vi "Hands Controller.vi"(8 "error in":errorcluster) -> ()   [LabVIEW 2017]
doc: "This VI executes continuously carrying out the current operation and responding to updates or new operations. It will often contain the timing or control code that is difficult to place directly in TeleOp. This VI generally opens all sensors and motors and isolates the rest of the robot code from knowing how the operations are carried out."
uses:
  <vilib>/Rock Robotics/WPI/Framework/Completion Status.ctl
  Hands Setpoints.ctl
  Hands Operations.ctl
  <vilib>/Rock Robotics/WPI/SafetyOutput/WPI_SafetyOutputConfigMenu.ctl
  <vilib>/Rock Robotics/SystemInterfaces/DIO/FPGA_DIOPWMChannel.ctl
  <vilib>/Rock Robotics/WPI/MotorControl/WPI_MotorControlOpen VictorSP.vi
  <vilib>/Rock Robotics/Network Tables/NT Write Boolean.vi
panel:
  in  "Slide 2":dbl(slide) scale=-0.8..0.8
  in  "Slide":dbl(slide) scale=-0.8..0.8
  out "Waveform Chart":dbl(graph)
  in  "Interactive Values":T1
  out "Current\nCmd":string
  in  "Buttons":cluster{"Execute Cmd":bool, "Abort Cmd":bool}
  out "Command Timing":cluster{"Start Time (ms)":u32, "Iterations":i32}
  out "Status":T3
  # "Tip: It may be helpful to observe inputs and sensor values.\nYou may also want to display tuning or debugging controls."
  # "Interactive Command: You may fill in the settings for a command\nand schedule it with the Execute button. You can observe and abort\nany command while fine tuning the code for the controller."
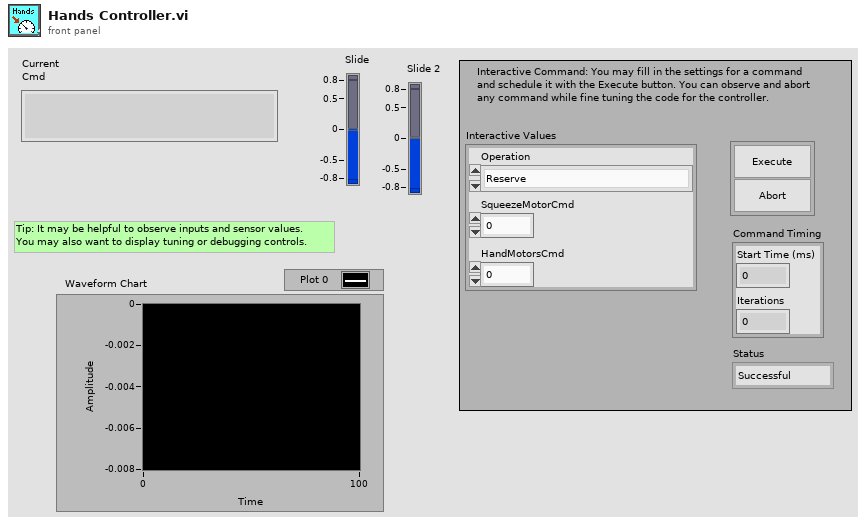
[diagram p1: front panel]
types:
  T1 = typedef "Hands Setpoints.ctl" = cluster{"Operation":T2, "SqueezeMotorCmd":dbl, "HandMotorsCmd":dbl}
  T2 = typedef "Hands Operations.ctl" = enum16{"Reserve", "Read Current", "Immediate"}
  T3 = typedef "Completion Status.ctl" = enum16{"Successful", "Aborted", "Incomplete"}
  T4 = typedef "FPGA_DIOPWMChannel.ctl" = enum8{"PWM 0", "PWM 1", "PWM 2", "PWM 3", "PWM 4", "PWM 5", "PWM 6", "PWM 7", "PWM 8", "PWM 9", "PWM MXP 0", "PWM MXP 1", "PWM MXP 2", "PWM MXP 3", "PWM MXP 4", "PWM MXP 5", "PWM MXP 6", "PWM MXP 7", "PWM MXP 8", "PWM MXP 9", "Invalid"}
  T5 = typedef "WPI_SafetyOutputConfigMenu.ctl" = enum16{"Enable", "Disable"}
  T6 = typedef "WPI_MotorControlDeviceRef.ctl" = cluster{"DeviceStatus":errorcluster, "Type":T7, "PWM":cluster{"PWM Channel":T4, "DeadBand":T8}, "CAN":cluster{"Device Number":u8, "SetOutput VI Ref":variant, "GetOutput VI Ref":variant, "Enable VI Ref":variant, "Disable VI Ref":variant, "Data":variant}, "Invert":bool, "DIO PWM":cluster{"PWM \"Enable\" Channel":T4, "DIOChannel":T9, "PWM Rate":dbl}}
  T7 = typedef "WPI_MotorControlType.ctl" = enum16{"PWM", "CAN", "DIO PWM"}
  T8 = typedef "WPI_PWMDeadband.ctl" = cluster{"Name":string, "maxPositivePwm":i32, "minPositivePwm":i32, "centerPwm":i32, "maxNegativePwm":i32, "minNegativePwm":i32, "angularRange":u16}
  T9 = typedef "FPGA_DIOChannel.ctl" = enum8{"DIO 0", "DIO 1", "DIO 2", "DIO 3", "DIO 4", "DIO 5", "DIO 6", "DIO 7", "DIO 8", "DIO 9", "DIO MXP 0", "DIO MXP 1", "DIO MXP 2", "DIO MXP 3", "DIO MXP 4", "DIO MXP 5", "DIO MXP 6", "DIO MXP 7", "DIO MXP 8", "DIO MXP 9", "DIO MXP 10", "DIO MXP 11", "DIO MXP 12", "DIO MXP 13", "DIO MXP 14", "DIO MXP 15", "SPI Port CS1", "SPI Port CS2", "SPI Port CS3", "SPI Port MISO", "SPI Port MOSI", "Invalid"}
  T10 = typedef "Command Status Info.ctl" = cluster{"Name":string, "Status":T3, "notifier out":T11}
  T11 = typedef "Completion Notifier.ctl" = refnum<notifier>
  T12 = cluster{"Current Command":T1, "Command Timing":cluster{"Start Time (ms)":u32, "Iterations":i32}, "Command Arguments":cluster{"Command Info":T10, "Description":string, "Default Command":T1, "queue out":refnum<queue>, "Subsystem Name":string}}
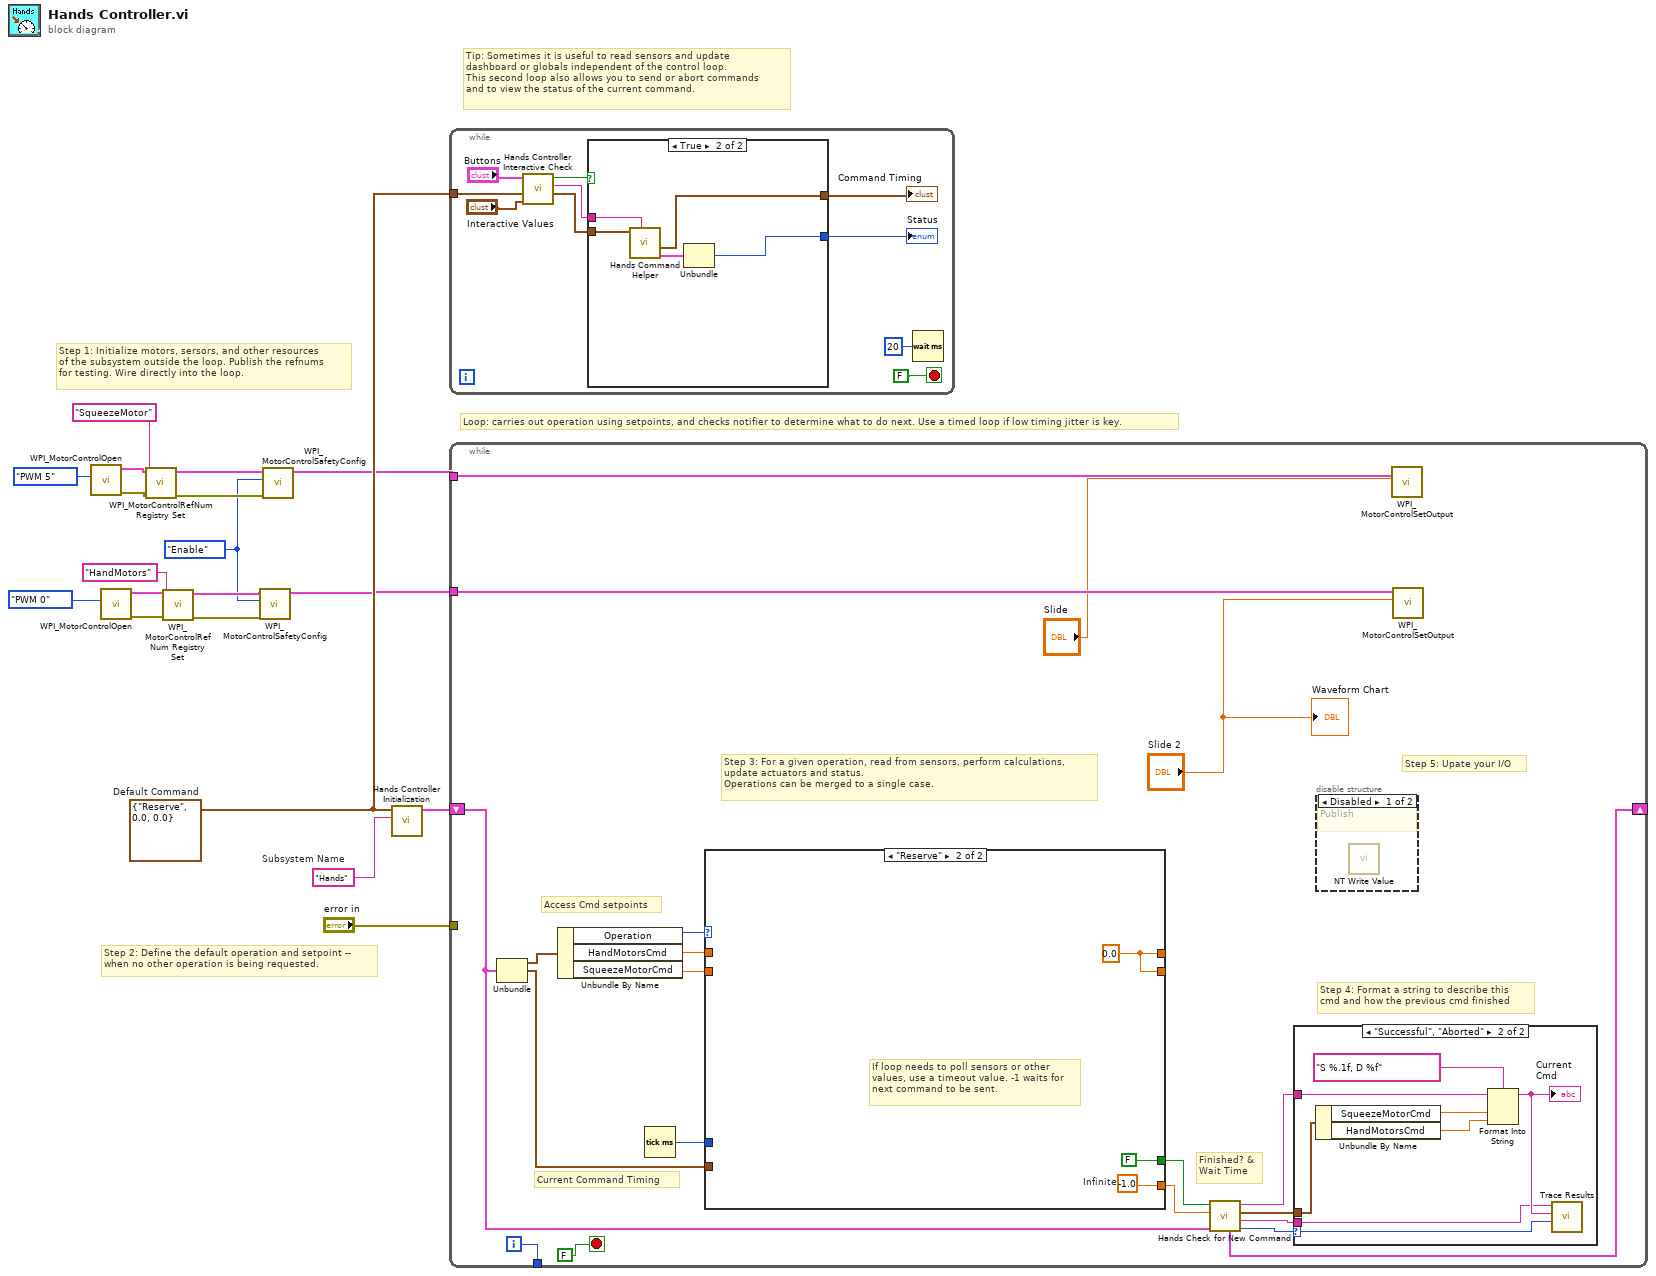
[diagram p0: block diagram]
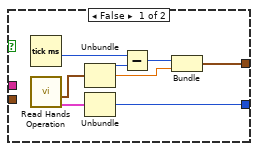
[diagram p2: hidden frame]
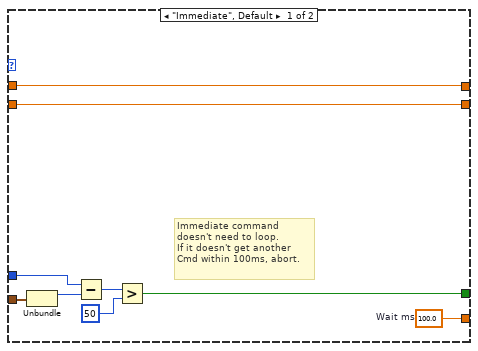
[diagram p5: hidden frame]
diagram:
  w1 = WPI_SafetyOutputConfigMenu."Enable" ("mode")
  w16 = T1 {"Operation"=enum."Reserve", "SqueezeMotorCmd"=0.0, "HandMotorsCmd"=0.0}  # Default Command
  w17 = "Hands"  # Subsystem Name
  # "Tip: Sometimes it is useful to read sensors and update\ndashboard or globals independent of the control loop.\nThis second loop also allows you to send or abort commands\nand to view the status of the current command."
  # "Step 2: Define the default operation and setpoint --\nwhen no other operation is being requested."
  # "Step 1: Initialize motors, sersors, and other resources\nof the subsystem outside the loop. Publish the refnums\nfor testing. Wire directly into the loop."
  # "Loop: carries out operation using setpoints, and checks notifier to determine what to do next. Use a timed loop if low timing jitter is key."
  n1 = call-poly <vilib>:"WPI_MotorControlOpen.vi"("PWM Channel"=FPGA_DIOPWMChannel."PWM 5") -> ("error out"=w7:errorcluster, "MotorControlDeviceRef"=w8:T6)  [unwired: 9 in]
  n2 = call-poly <vilib>:"WPI_MotorControlOpen.vi"("PWM Channel"=FPGA_DIOPWMChannel."PWM 0") -> ("error out"=w12:errorcluster, "MotorControlDeviceRef"=w10:T6)  [unwired: 9 in]
  n3 = call <vilib>:"WPI_MotorControlRefNum Registry Set.vi"("error in (no error)"=w7, "refnum name"="SqueezeMotor", "MotorControlDevRef"=w8) -> ("error out"=w4:errorcluster, "MotorControlDevRef"=w5:T6)  [unwired: 7 in]
  n4 = call <vilib>:"WPI_MotorControlRefNum Registry Set.vi"("error in (no error)"=w12, "refnum name"="HandMotors", "MotorControlDevRef"=w10) -> ("error out"=w13:errorcluster, "MotorControlDevRef"=w14:T6)  [unwired: 7 in]
  n5 = call <vilib>:"WPI_MotorControlSafetyConfig.vi"("error in (no error)"=w13, "mode"=w1, "MotorControlDevRef"=w14) -> ("MotorControlDevRef"=w15:T6)  [unwired: 7 in, 1 out]
  n6 = call <vilib>:"WPI_MotorControlSafetyConfig.vi"("error in (no error)"=w4, "mode"=w1, "MotorControlDevRef"=w5) -> ("MotorControlDevRef"=w3:T6)  [unwired: 7 in, 1 out]
  n7 = call "Hands Controller Initialization.vi"("Subsystem Name"=w17, "Default Command"=w16) -> ("Current Command"=w18:T12)  [unwired: 9 in]
  n8 = while {
    tunnel: w16 -> [w26]
    stop <- FALSE stop-if-true
    n9 = call "Hands Controller Interactive Check.vi"("Interactive Command in"="Interactive Values", "Default Command"=w26, "Buttons"="Buttons") -> ("Interactive Command out"=w23:T1, "Trace String"=w24:string, "Schedule"=w25:bool)  [unwired: 6 in]
    n10 = case shown="True" w25 {
      tunnel: [w37 w42] -> w22
      tunnel: w23 -> [_ w40]
      tunnel: [w33 w38] -> w21
      tunnel: w24 -> [_ w41]
      frame False {
        n11 = Tick Count (ms)() -> (millisecond timer value=w32:u32)
        n12 = call "Read Hands Operation.vi"() -> ("Command Info"=w30:T10, "SubSystem Data"=w31:T1)  [unwired: 9 in, 1 out]
        n13 = Unbundle(w31) -> ("Operation"=w36:T2, "SqueezeMotorCmd"=w34:dbl)  [unwired: 1 out]
        n14 = Unbundle(w30) -> ("Status"=w37:T3)  [unwired: 2 out]
        n15 = Subtract(x=w32, y=w36) -> (x-y=w35:u32)
        n16 = Bundle(w35, "SqueezeMotorCmd"=w34) -> (w33:cluster{u32, "SqueezeMotorCmd":dbl})  [unwired: 1 in]
      }
      frame True {
        n17 = call "Hands Command Helper.vi"("Description"=w41, "SubSystem Data"=w40) -> ("Command Info Out"=w39:T10, "Command Timing"=w38:cluster{"Start Time (ms)":u32, "Iterations":i32})  [unwired: 7 in, 1 out]
        n18 = Unbundle(w39) -> ("Status"=w42:T3)  [unwired: 2 out]
      }
    }
    "Status" <- w22
    "Command Timing" <- w21
    n19 = Wait (ms)(milliseconds to wait=u32 20) -> ()  [unwired: 1 out]
  }
  n20 = while {
    shift-right: [w54] -> _
    shift-left: w18 -> [w47]
    tunnel: [w61] -> _
    tunnel: "error in" -> [_]
    tunnel: w15 -> [w45]
    tunnel: w3 -> [w46]
    i -> [w61]
    stop <- FALSE stop-if-true
    # "Step 5: Upate your I/O"
    # "Step 4: Format a string to describe this\ncmd and how the previous cmd finished"
    # "Current Command Timing"
    # "Access Cmd setpoints"
    # "Finished? &\nWait Time"
    # "Step 3: For a given operation, read from sensors, perform calculations,\nupdate actuators and status.\nOperations can be merged to a single case."
    n21 = Unbundle(w47) -> ("Current Command"=w60:T1, "Command Timing"=w56:cluster{"Start Time (ms)":u32, "Iterations":i32})  [unwired: 1 out]
    n22 = Unbundle By Name(w60) -> ("Operation"=w59:T2, "HandMotorsCmd"=w58:dbl, "SqueezeMotorCmd"=w55:dbl)
    n23 = Tick Count (ms)() -> (millisecond timer value=w57:u32)
    n24 = case shown="\"Reserve\"" w59 {
      tunnel: [w79 w82] -> w52
      tunnel: [w73 FALSE ("ignore previous (F)")] -> w53
      tunnel: w56 -> [w75 _]
      tunnel: w58 -> [w72 _]
      tunnel: w57 -> [w74 _]
      tunnel: w55 -> [w71 _]
      tunnel: [w72 w80] -> _
      tunnel: [w71 w80] -> _
      frame "Immediate", Default {
        w79 = 100.0  # Wait ms
        # "Immediate command\ndoesn't need to loop.\nIf it doesn't get another\nCmd within 100ms, abort."
        n25 = Unbundle(w75) -> ("Start Time (ms)"=w78:u32)  [unwired: 1 out]
        n26 = Subtract(x=w74, y=w78) -> (x-y=w77:u32)
        n27 = Greater?(x=w77, y=u8 50 ("Left Motor")) -> (0:w73:bool)
      }
      frame "Reserve" {
        w80 = 0.0 ("HandMotorsCmd")
        w82 = -1.0  # Infinite
        # "If loop needs to poll sensors or other\nvalues, use a timeout value. -1 waits for\nnext command to be sent."
      }
    }
    n28 = call "Hands Check for New Command.vi"("Current Command"=w47, "Wait time (ms)"=w52, "Finished?"=w53) -> ("Completion"=w48:T3, "Subsystem Name"=w49:string, "Current Command"=w50:T1, "Initial Trace String"=w51:string, "NextCommand"=w54:T12)  [unwired: 4 in]
    n29 = case shown="\"Successful\", \"Aborted\"" w48 {
      selector: w48 -> [_ w70]
      tunnel: w51 -> [_ w66]
      tunnel: w50 -> [_ w67]
      tunnel: w49 -> [_ w63]
      frame "Incomplete", Default {
        # "Continuing current command"
      }
      frame "Successful", "Aborted" {
        # "Report and setup for next command"
        n30 = Unbundle By Name(w67) -> ("SqueezeMotorCmd"=w69:dbl, "HandMotorsCmd"=w64:dbl)
        n31 = Format Into String(format string="S %.1f, D %f", initial string=w66, w69, w64) -> (resulting string=w65:string)  [unwired: 1 in, 1 out]
        "Current\nCmd" <- w65
        n32 = call <vilib>:"Trace Results.vi"("Status of previous command"=w70, "Description"=w65, "Subsystem"=w63) -> ()  [unwired: 9 in]
      }
    }
    n33 = disable-structure shown="Disabled" {
      frame Disabled {
        # "Publish"
        n34 = call-poly <vilib>:"NT Write Value.vi"() -> ()  [unwired: 11 in, 1 out]
      }
      frame Enabled {
      }
    }
    n35 = call <vilib>:"WPI_MotorControlSetOutput.vi"("Output"="Slide", "MotorControlDevRef"=w46) -> ()  [unwired: 7 in, 3 out]
    n36 = call <vilib>:"WPI_MotorControlSetOutput.vi"("Output"="Slide 2", "MotorControlDevRef"=w45) -> ()  [unwired: 7 in, 3 out]
    "Waveform Chart" <- "Slide 2"
  }
